vi "controlActorSelection.vi"(7 "set":bool, 8 "error in":errorcluster, 9 "Positioner in":string, 10 "axis":u8(ring) items=["1", "2", "3"], 11 "connection ID":i32) -> (0 "error out":errorcluster, 1 "Positioner out":string, 2 "axis out":u8, 3 "connection ID":i32, 4 "allPositioners":string[](array[string]))   [LabVIEW 2016]
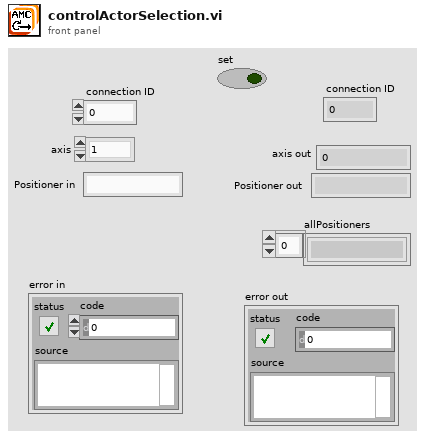
[diagram p1: front panel]
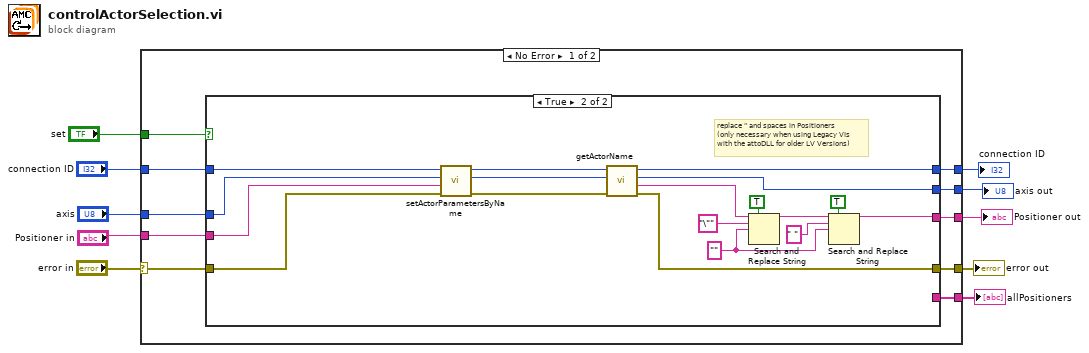
[diagram p0: block diagram]
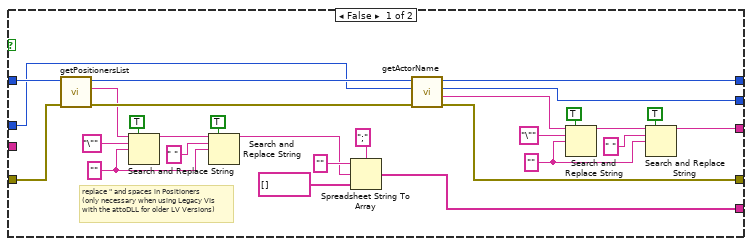
[diagram p2: hidden frame]
diagram:
  n1 = case shown="No Error" "error in" {
    selector: "error in" -> [w18 w68]
    tunnel: "axis" -> [w16 w69]
    tunnel: [w17 w68] -> w10
    tunnel: [w15 w69] -> w9
    tunnel: "Positioner in" -> [w14 w67]
    tunnel: [w19 w70] -> w7
    tunnel: "connection ID" -> [w20 w70]
    tunnel: "set" -> [w13 _]
    tunnel: [w12 w67] -> w3
    tunnel: [w11 _] -> w2
    frame No Error {
      n2 = case shown="True" w13 {
        tunnel: w20 -> [w42 w66]
        tunnel: [w48 w61] -> w19
        tunnel: w18 -> [w39 w65]
        tunnel: [w46 w59] -> w17
        tunnel: w16 -> [w40 w64]
        tunnel: [w47 w57] -> w15
        tunnel: w14 -> [_ w63]
        tunnel: [w21 w49] -> w12
        tunnel: [w37 _] -> w11
        frame False {
          w25 = "" ("replace string (\"\")")
          w31 = "" ("replace string (\"\")")
          # "replace \" and spaces in Positioners\n(only necessary when using Legacy VIs\nwith the attoDLL for older LV Versions)"
          n3 = call "getPositionersList.vi"("error in"=w39, "connection ID"=w42) -> ("error out"=w38:errorcluster, "PositionersList"=w36:string, "connection ID"=w41:i32)  [unwired: 7 in]
          n4 = Search and Replace String(replace all?=TRUE ("replace all? (F)"), input string=w36, search string="\"", replace string=w31) -> (result string=w35:string)  [unwired: 4 in, 3 out]
          n5 = Search and Replace String(replace all?=TRUE ("replace all? (F)"), input string=w35, search string=" ", replace string=w31) -> (result string=w34:string)  [unwired: 4 in, 3 out]
          n6 = Spreadsheet String To Array(delimiter (Tab)=";", format string="", spreadsheet string=w34, array type (2D Dbl)=string[] []) -> (array=w37:string[])
          n7 = call "getActorName.vi"("error in"=w38, "axis"=w40, "connection ID"=w41) -> ("error out"=w46:errorcluster, "actor_name"=w22:string, "axis_out"=w47:i32, "connection ID"=w48:i32)  [unwired: 5 in]
          n8 = Search and Replace String(replace all?=TRUE ("replace all? (F)"), input string=w22, search string="\"", replace string=w25) -> (result string=w28:string)  [unwired: 4 in, 3 out]
          n9 = Search and Replace String(replace all?=TRUE ("replace all? (F)"), input string=w28, search string=" ", replace string=w25) -> (result string=w21:string)  [unwired: 4 in, 3 out]
        }
        frame True {
          w53 = "" ("replace string (\"\")")
          # "replace \" and spaces in Positioners\n(only necessary when using Legacy VIs\nwith the attoDLL for older LV Versions)"
          n10 = call "setActorParametersByName.vi"("error in"=w65, "actorname"=w63, "axis"=w64, "connection ID"=w66) -> ("error out"=w60:errorcluster, "axis_out"=w58:i32, "connection ID"=w62:i32)  [unwired: 5 in]
          n11 = call "getActorName.vi"("error in"=w60, "axis"=w58, "connection ID"=w62) -> ("error out"=w59:errorcluster, "actor_name"=w50:string, "axis_out"=w57:i32, "connection ID"=w61:i32)  [unwired: 5 in]
          n12 = Search and Replace String(replace all?=TRUE ("replace all? (F)"), input string=w50, search string="\"", replace string=w53) -> (result string=w56:string)  [unwired: 4 in, 3 out]
          n13 = Search and Replace String(replace all?=TRUE ("replace all? (F)"), input string=w56, search string=" ", replace string=w53) -> (result string=w49:string)  [unwired: 4 in, 3 out]
        }
      }
    }
    frame Error {
    }
  }
  "error out" <- w10
  "axis out" <- w9
  "connection ID" <- w7
  "Positioner out" <- w3
  "allPositioners" <- w2
